vi "Exercise 3.1 - Simulated.vi"() -> ()   [LabVIEW 2012]
panel:
  out "Frequency":dbl
  out "Amplitude":dbl
  in  "stop":bool
  in  "Frequency In":dbl(knob) scale=0.0..10.0
  out "Waveform Chart":dynamicdata(graph)
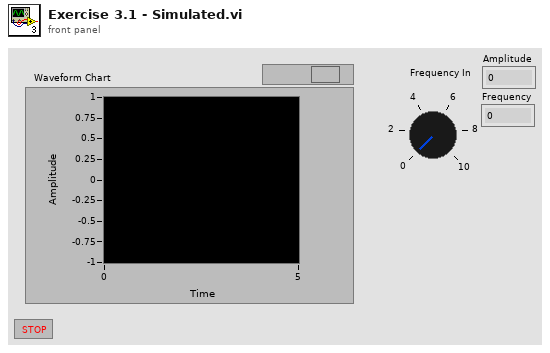
[diagram p1: front panel]
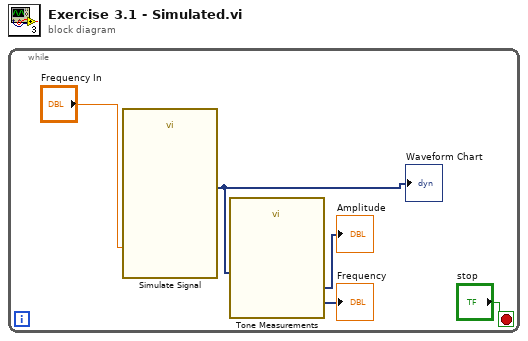
[diagram p0: block diagram]
diagram:
  n1 = while {
    stop <- "stop" stop-if-true
    n2 = call "Simulate Signal"("Frequency"="Frequency In") -> ("Sine"=w1:dynamicdata)  [unwired: 13 in, 1 out]
    "Waveform Chart" <- w1
    n3 = call "Tone Measurements"("Signals"=w1) -> ("Frequency"=→"Frequency":dynamicdata, "Amplitude"=→"Amplitude":dynamicdata)  [unwired: 8 in, 1 out]
  }
